vi "FGV_Error.vi"(8 "error_in_loop":errorcluster, 11 "Estado":enum16{"Set", "Get"}(ring)) -> (0 "error out":errorcluster)   [LabVIEW 2026]
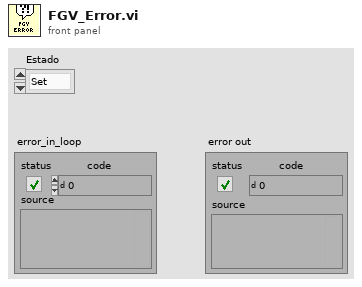
[diagram p1: front panel]
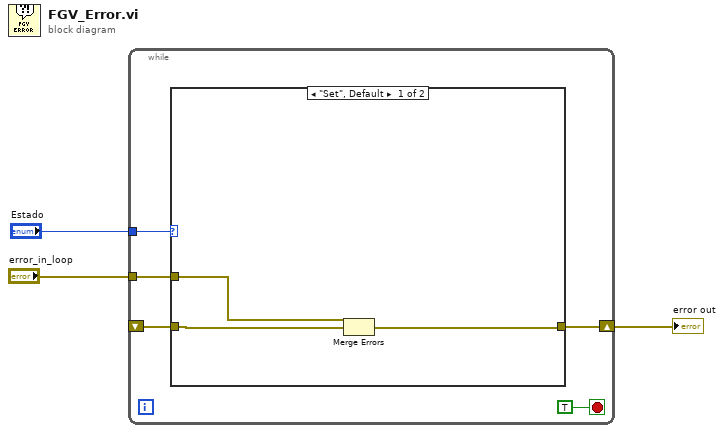
[diagram p0: block diagram]
diagram:
  n1 = while {
    tunnel: "Estado" -> [w8]
    shift-right: [w7] -> w2
    shift-left: _ -> [w6]
    tunnel: "error_in_loop" -> [w4]
    stop <- TRUE stop-if-true
    n2 = case shown="\"Set\", Default" w8 {
      tunnel: [w10 w12] -> w7
      tunnel: w6 -> [w9 w12]
      tunnel: w4 -> [w11 _]
      frame "Set", Default {
        n3 = Merge Errors(w11, w9) -> (w10:errorcluster)
      }
      frame "Get" {
      }
    }
  }
  "error out" <- w2
